vi "수신.vi"() -> ()   [LabVIEW 2023]
panel:
  in  "stop":bool
  out "data out":string
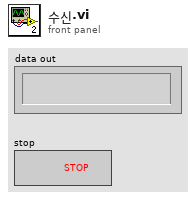
[diagram p1: front panel]
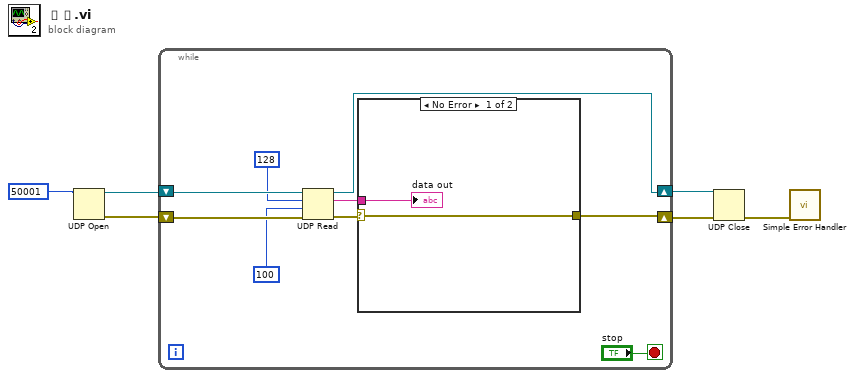
[diagram p0: block diagram]
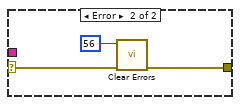
[diagram p2: hidden frame]
diagram:
  n1 = UDP Open(11:u16 50001 ("port")) -> (port=w6:refnum<k16>, 0:w5:errorcluster)  [unwired: 4 in, 1 out]
  n2 = while {
    shift-right: [w14] -> w4
    shift-left: w5 -> [w10]
    shift-right: [w13] -> w2
    shift-left: w6 -> [w12]
    stop <- "stop" stop-if-true
    n3 = UDP Read(connection ID=w12, max size (548)=128, timeout ms (25000)=100, 8:w10) -> (data out=w11:string, error out=w15:errorcluster, 3:w13:refnum<k16>)  [unwired: 2 out]
    n4 = case shown="No Error" w15 {
      selector: w15 -> [w17 w20]
      tunnel: [w17 w19] -> w14
      tunnel: w11 -> [w16 _]
      frame No Error {
        "data out" <- w16
      }
      frame Error {
        n5 = call <vilib>:"Clear Errors.vi"("error in (no error)"=w20, "specific error code to clear (0: all)"=56) -> ("error out"=w19:errorcluster)  [unwired: 4 in, 1 out]
      }
    }
  }
  n6 = UDP Close(connection ID=w2, 8:w4) -> (error out=w3:errorcluster)  [unwired: 1 out]
  n7 = call <vilib>:"Simple Error Handler.vi"("error in (no error)"=w3) -> ()  [unwired: 4 in, 5 out]
